vi "generate_ramp.vi"(2 "error in (no error)":errorcluster, 3 "VISA Refnum in":refnum<visa-resource-name>) -> (0 "error out":errorcluster, 1 "VISA Refnum out":refnum<visa-resource-name>)   [LabVIEW 2013]
uses:
  <vilib>/Analysis/1siggen.llb/Ramp Pattern by Samples.vi
  <vilib>/Analysis/NI_AALBase.lvlib
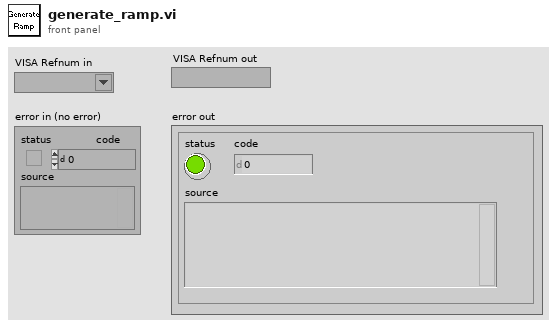
[diagram p1: front panel]
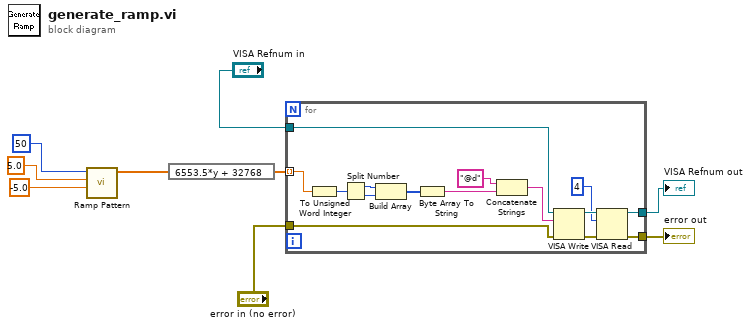
[diagram p0: block diagram]
diagram:
  n1 = call-poly <vilib>:"Ramp Pattern.vi"("start"=-5.0, "end"=5.0, "samples"=50) -> ("Ramp Pattern"=w6:dbl[])  [unwired: 7 in, 1 out]
  n2 = expression code="6553.5*y + 32768"(w6) -> (w4:dbl[])
  n3 = for {
    tunnel: w4 -> [w14] mode=indexing
    tunnel: [w13] -> w7
    tunnel: [w12] -> w8
    tunnel: "VISA Refnum in" -> [w11]
    tunnel: "error in (no error)" -> [w10]
    n4 = To Unsigned Word Integer(number=w14) -> (unsigned 16bit integer=w23:u16)
    n5 = Split Number(x=w23) -> (hi(x)=w20:u8, lo(x)=w21:u8)
    n6 = Build Array(w20, w21) -> (w24:u8[])
    n7 = Byte Array To String(unsigned byte array=w24) -> (string=w22:string)
    n8 = Concatenate Strings("@d" ("write buffer"), w22) -> (w16:string)
    n9 = VISA Write(VISA resource name=w11, write buffer=w16, error in (no error)=w10) -> (VISA resource name out=w18:refnum<visa-resource-name>, error out=w19:errorcluster)  [unwired: 1 out]
    n10 = VISA Read(VISA resource name=w18, byte count=u32 4, error in (no error)=w19) -> (VISA resource name out=w13:refnum<visa-resource-name>, error out=w12:errorcluster)  [unwired: 2 out]
  }
  "VISA Refnum out" <- w7
  "error out" <- w8
